vi "SVPO Power in Band (1 Ch SGL Spectrum).vi"(0 "spectrum [EU^2 rms]":cluster{"x0":dbl, "dx":dbl, "magnitude":sgl[]}={"x0"=0.0, "dx"=1.0, "magnitude"=[]} {"magnitude" format="%.2f"; "dx" format="%.2f"; "x0" format="%.2f"}, 1 "range":cluster{"start":dbl, "stop":dbl}={"start"=0.0, "stop"=1000.0} {"stop" format="%.2f"; "start" format="%.2f"}, 4 "spectrum info":T1={"channel name"="", "description"="", "x-axis units"=0, "spectral info"={"spectrum type"=enum."Power [Magnitude^2]", "linear/dB"=enum."linear", "window"=0, "window size"=0, "FFT size"=0}, "engineering units"=0, "custom label"="", "dB reference [EU]"=0.0, "peak units"=enum."rms", "weighting filter"=0, "spectral density?"=FALSE, "unit label"="", "spectrum skewed?"=FALSE, "complimentary spectrum units"=enum."none"} {"x-axis units" items=["Time (s)"=0, "Frequency-CB (Hz)"=1, "Frequency-CPB (Hz)"=1248, "Frequency-Arbitrary (Hz)"=2357, "Quefrency (s)"=2, "Revolutions (rev)"=3, "Order"=4, "Speed (RPM)"=11, "Speed (rad/s)"=21, "Index"=65535]; "weighting filter" items=["Linear", "A-weighting", "B-weighting", "C-weighting", "ITU-R 468-4", "Dolby", "CCITT", "C-message", "Wb", "Wc", "Wd", "We", "Wf", "Wh", "Wj", "Wk", "Wm", "AES17 20 kHz lowpass", "AES17 40 kHz lowpass", "AES17 20 kHz highpass", "AES17 40 kHz highpass"]; "dB reference [EU]" format="%.2f"; "engineering units" items=["custom..."=0, "V"=1, "A"=21, "C"=30, "pC"=31, "s"=32, "-"=29, "Pa"=2, "N"=20, "g"=3, "m/s^2"=4, "m/s"=5, "m"=6, "mm/s"=12, "mm"=13, "micron/s"=14, "micron"=15, "in/s^2"=7, "in/s"=8, "in"=9, "mil/s"=10, "mil"=11, "rad/s^2"=16, "rad/s"=17, "rad"=18, "deg/s^2"=26, "deg/s"=27, "deg"=28, "RPM"=22, "cycle/s^2"=23, "Hz"=24, "cycle"=25, "strain"=19]; "spectral info"."window" items=["None "=0, "Hanning"=1, "Hamming"=2, "Blackman-Harris"=3, "Exact Blackman"=4, "Blackman"=5, "Flat Top"=6, "4 Term B-Harris "=7, "7 Term B-Harris"=8, "Low Sidelobe"=9, "Force - Exponential"=10, "Gaussian"=62]}) -> (14 "power in band [EU^2 rms]":dbl=nan format="%.2f")   [LabVIEW 2017, in "VibrationAnalysisFunctions.lvlib"]
doc: "Computes the aggregate power of a linear-scale power spectrum within the specified frequency <B>range</B> of the input spectrum. Use this VI on embedded targets that have limited computational resources. Wire data to the <B>spectrum [EU^2 rms]</B> input to determine the polymorphic instance to use or manually select the instance."
uses:
  <vilib>/addons/InsightCM/Utilities/Analysis/Vibration/VibrationAnalysisFunctions.lvlib
  <vilib>/addons/_NISVFA/_Shared subVIs/Controls/svc_Spectrum Info.ctl
  <vilib>/addons/_NISVFA/_Shared subVIs/Controls/svc_X-Axis Units.ctl
  <vilib>/addons/_NISVFA/_Shared subVIs/Controls/svc_Spectrum Type.ctl
  <vilib>/addons/_NISVFA/_Shared subVIs/Controls/svc_Engineering Units Text Ring.ctl
  <vilib>/addons/_NISVFA/_Shared subVIs/Controls/svc_Weighting Filter Text Ring.ctl
  <vilib>/addons/_NISVFA/_Shared subVIs/Controls/svc_Complimentary Spectrum Units.ctl
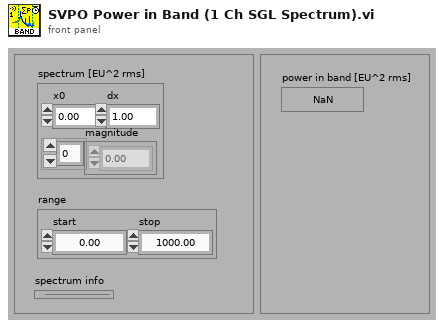
[diagram p1: front panel]
types:
  T1 = typedef "svc_Spectrum Info.ctl" = cluster{"channel name":string, "description":string, "x-axis units":T2, "spectral info":cluster{"spectrum type":T3, "linear/dB":enum16{"linear", "dB"}, "window":u16, "window size":i32, "FFT size":i32}, "engineering units":T4, "custom label":string, "dB reference [EU]":dbl, "peak units":enum16{"rms", "peak", "peak-peak"}, "weighting filter":T5, "spectral density?":bool, "unit label":string, "spectrum skewed?":bool, "complimentary spectrum units":T6}
  T2 = typedef "svc_X-Axis Units.ctl" = u16
  T3 = typedef "svc_Spectrum Type.ctl" = enum16{"FFT Spectrum [complex]", "Amplitude [Magnitude]", "Power [Magnitude^2]", "Cross Spectrum [complex]", "Frequency Response [Complex]"}
  T4 = typedef "svc_Engineering Units Text Ring.ctl" = u16
  T5 = typedef "svc_Weighting Filter Text Ring.ctl" = u16
  T6 = typedef "svc_Complimentary Spectrum Units.ctl" = enum16{"none", "radians", "degrees", "cycles", "imaginary"}
  T7 = typedef "NI_AALPro.lvlib/windowTd.ctl" = u32
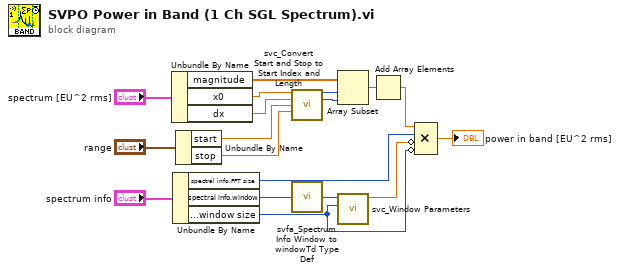
[diagram p0: block diagram]
diagram:
  n1 = Unbundle By Name("spectrum [EU^2 rms]") -> ("magnitude"=w11:sgl[], "x0"=w1:dbl, "dx"=w13:dbl)
  n2 = Unbundle By Name("spectrum info") -> ("spectral info.FFT size"=w12:i32, "spectral info.window"=w17:u16, "spectral info.window size"=w16:i32)
  n3 = Unbundle By Name("range") -> ("start"=w8:dbl, "stop"=w10:dbl)
  n4 = call <vilib>:"svc_Convert Start and Stop to Start Index and Length.vi"("f0"=w1, "df"=w13, "start frequency"=w8, "stop frequency"=w10) -> ("start index"=w4:i32, "band length"=w3:i32)  [unwired: 8 in, 2 out]
  n5 = call <vilib>:"svfa_Spectrum Info Window to windowTd Type Def.vi"("window"=w17) -> ("window"=w2:T7)  [unwired: 4 in]
  n6 = Array Subset(array=w11, index=w4, length=w3) -> (w6:sgl[])
  n7 = call <vilib>:"svc_Window Parameters.vi"("window size"=w16, "window"=w2) -> ("ENBW"=w7:dbl)  [unwired: 6 in, 3 out]
  n8 = Add Array Elements(numeric array=w6) -> (sum=w5:sgl)
  n9 = Compound Arithmetic op=MULTIPLY(w5, w12, invert w7, invert w16) -> (→"power in band [EU^2 rms]":dbl)
